vi "SSL Data Receiver.vi"(11 "SSL Data 2":refnum<vi>) -> (1 "IA flags":T1, 2 "SSL RefBox":T1, 3 "SSL Vision":T1)   [LabVIEW 2017]
uses:
  <extravilib>/ChannelInstances/Lossy Stream-a[.](u8)/)Channel.ctl
  Control/SSL Data Control.ctl
  Control/SSL UDP Address.ctl
  Control/File Player.ctl
  <extravilib>/ChannelInstances/Lossy Stream-a[.](u8)/Write With Abort.vi
  <extravilib>/ChannelInstances/Lossy Stream-a[.](u8)/Endpoint.vi
  <extravilib>/ChannelInstances/Lossy Stream-a[.](u8)/Instantiate.vi
  <extravilib>/ChannelInstances/Stream-a[.](u8)/Instantiate.vi
  <extravilib>/ChannelInstances/Lossy Stream-a[.](u8)/)Channel.vi
  <extravilib>/ChannelInstances/Lossy Stream-a[.](u8).lvlib
panel:
  in  "SSL UDP SOS RX":refnum<vi>
  out "error out 2":errorcluster
  in  "Boolean 2":refnum<vi>
  in  "Cluster in":refnum<vi>
  in  "RefBox UDP RX":refnum<vi>
  in  "SSL UDP RX":refnum<vi>
  out "error out":errorcluster
  out "error out 4":errorcluster
  out "error out":errorcluster
  # "UDP"
  # "LOG"
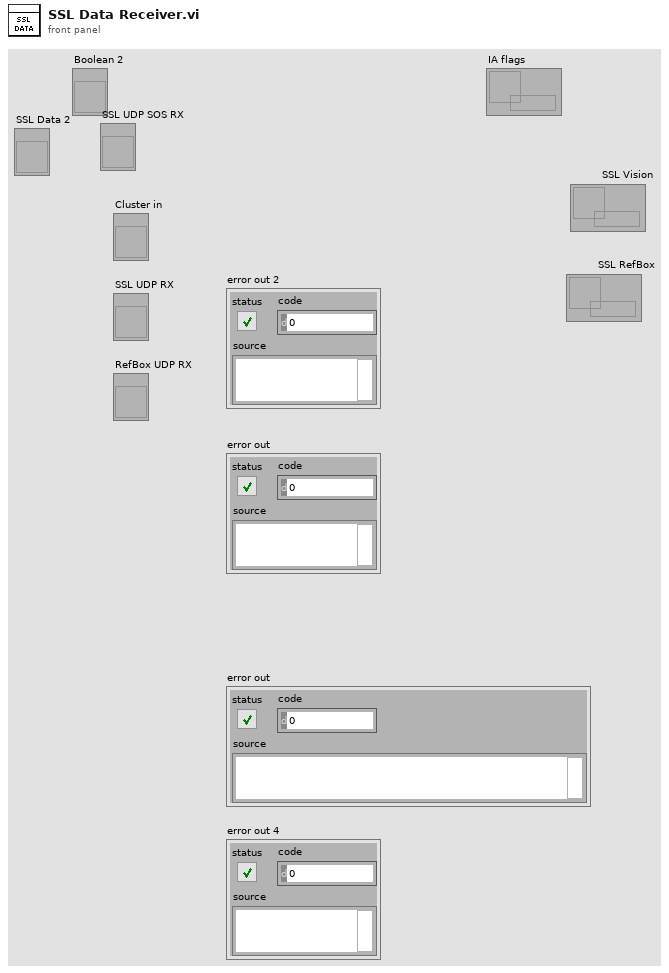
[diagram p1: front panel]
types:
  T1 = typedef "Lossy Stream-a[.](u8).lvlib/)Channel.ctl" = refnum<queue>
  T2 = typedef "Stream-a[.](u8).lvlib/)Channel.ctl" = refnum<queue>
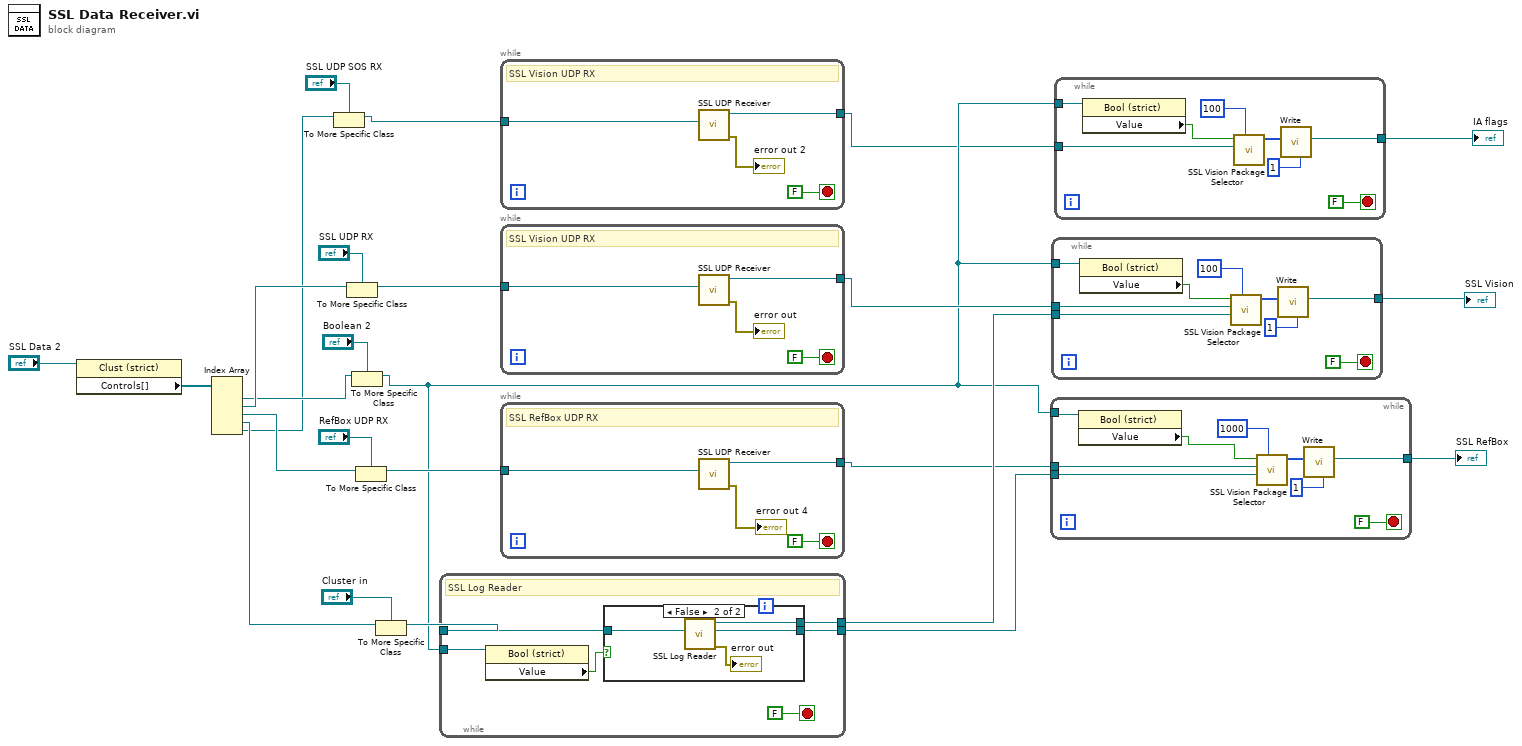
[diagram p0: block diagram]
diagram:
  n1 = property on="Property Node" class="Clust (strict)"(reference="SSL Data 2") -> ("Controls[]"=w19:refnum<vi>[])  [unwired: 1 in, 2 out]
  n2 = Index Array(array=w19) -> (element #1=w7:refnum<vi>, element #2=w16:refnum<vi>, element #3=w13:refnum<vi>, element #4=w10:refnum<vi>, element #5=w1:refnum<vi>)  [unwired: 5 in]
  n3 = To More Specific Class(target class="SSL UDP SOS RX", reference=w1) -> (specific class reference=w5:refnum<vi>)  [unwired: 1 in, 1 out]
  n4 = To More Specific Class(target class="SSL UDP RX", reference=w16) -> (specific class reference=w17:refnum<vi>)  [unwired: 1 in, 1 out]
  n5 = To More Specific Class(target class="Boolean 2", reference=w7) -> (specific class reference=w4:refnum<vi>)  [unwired: 1 in, 1 out]
  n6 = To More Specific Class(target class="RefBox UDP RX", reference=w13) -> (specific class reference=w15:refnum<vi>)  [unwired: 1 in, 1 out]
  n7 = To More Specific Class(target class="Cluster in", reference=w10) -> (specific class reference=w12:refnum<vi>)  [unwired: 1 in, 1 out]
  n8 = while {
    tunnel: [w29] -> w22
    tunnel: [w30] -> w24
    tunnel: w12 -> [w28]
    tunnel: w4 -> [w27]
    stop <- FALSE stop-if-true
    # "SSL Log Reader"
    n9 = property class="Bool (strict)"(reference=w27) -> ("Value"=w26:bool)  [unwired: 1 in, 2 out]
    n10 = case shown="False" w26 {
      tunnel: [_ w34] -> w30
      tunnel: [_ w33] -> w29
      tunnel: w28 -> [_ w32]
      frame True {
      }
      frame False {
        n11 = call "SSL Log Reader.vi"("Cluster 2"=w32) -> ("error out"=→"error out":errorcluster, "channel 2"=w33:T2, "Channel out"=w34:T2)  [unwired: 7 in, 1 out]
      }
    }
  }
  n12 = while {
    tunnel: [w39] -> w3
    tunnel: w5 -> [w36]
    stop <- FALSE stop-if-true
    # "SSL Vision UDP RX"
    n13 = call "SSL UDP Receiver.vi"("SSL UDP Receiver 2"=w36) -> ("error out"=→"error out 2":errorcluster, "Channel out"=w39:T1)  [unwired: 9 in]
  }
  n14 = while {
    tunnel: [w43] -> w25
    tunnel: w17 -> [w40]
    stop <- FALSE stop-if-true
    # "SSL Vision UDP RX"
    n15 = call "SSL UDP Receiver.vi"("SSL UDP Receiver 2"=w40) -> ("error out"=→"error out":errorcluster, "Channel out"=w43:T1)  [unwired: 9 in]
  }
  n16 = while {
    tunnel: [w45] -> w23
    tunnel: w15 -> [w44]
    stop <- FALSE stop-if-true
    # "SSL RefBox UDP RX"
    n17 = call "SSL UDP Receiver.vi"("SSL UDP Receiver 2"=w44) -> ("error out"=→"error out 4":errorcluster, "Channel out"=w45:T1)  [unwired: 9 in]
  }
  n18 = while {
    tunnel: w23 -> [w56]
    tunnel: w22 -> [w55]
    tunnel: [w52] -> w21
    tunnel: w4 -> [w49]
    stop <- FALSE stop-if-true
    n19 = property class="Bool (strict)"(reference=w49) -> ("Value"=w50:bool)  [unwired: 1 in, 2 out]
    n20 = call "SSL Vision Package Selector.vi"("timeout in ms (-1)"=1000, "channel in"=w55, "Channel in"=w56, "Modo"=w50) -> ("element"=w53:u8[])  [unwired: 7 in]
    n21 = call <extravilib>:"Write.vi"("size (1)"=1, "element"=w53) -> ("channel"=w52:T1)  [unwired: 7 in, 2 out]
  }
  "SSL RefBox" <- w21
  n22 = while {
    tunnel: w25 -> [w65]
    tunnel: w24 -> [w64]
    tunnel: [w61] -> w20
    tunnel: w4 -> [w59]
    stop <- FALSE stop-if-true
    n23 = property class="Bool (strict)"(reference=w59) -> ("Value"=w58:bool)  [unwired: 1 in, 2 out]
    n24 = call "SSL Vision Package Selector.vi"("timeout in ms (-1)"=100, "channel in"=w64, "Channel in"=w65, "Modo"=w58) -> ("element"=w62:u8[])  [unwired: 7 in]
    n25 = call <extravilib>:"Write.vi"("size (1)"=1, "element"=w62) -> ("channel"=w61:T1)  [unwired: 7 in, 2 out]
  }
  "SSL Vision" <- w20
  n26 = while {
    tunnel: w3 -> [w73]
    tunnel: [w70] -> w2
    tunnel: w4 -> [w68]
    stop <- FALSE stop-if-true
    n27 = property class="Bool (strict)"(reference=w68) -> ("Value"=w67:bool)  [unwired: 1 in, 2 out]
    n28 = call "SSL Vision Package Selector.vi"("timeout in ms (-1)"=100, "Channel in"=w73, "Modo"=w67) -> ("element"=w71:u8[])  [unwired: 8 in]
    n29 = call <extravilib>:"Write.vi"("size (1)"=1, "element"=w71) -> ("channel"=w70:T1)  [unwired: 7 in, 2 out]
  }
  "IA flags" <- w2
